vi "Start Personal Log.vi"(8 "error in (no error)":errorcluster, 11 "Father of all uServices in":refnum<class "Father of all uServices.lvclass">) -> (0 "error out":errorcluster, 3 "Father of all uServices out":refnum<class "Father of all uServices.lvclass">)   [LabVIEW 2026, in "TALOS.lvlib" / "Father of all uServices.lvlib" / "Father of all uServices.lvclass"]
uses:
  Father of all uServices.lvclass
  C:/LabVIEW Code/TALOS/talos/Ancestor/Ancestor/Ancestor.lvclass
  Ancestor/Ancestor/Ancestor.lvclass/Ancestor.ctl
  Father of all uServices.lvclass/Father of all uServices.ctl
  Support VIs/Generate Error.vi
  FGV/Error Memory/Get Error Description.vi
  Support VIs/Get PC name.vi
  Support VIs/Get Class Name.vi
  <vilib>/Utility/error.llb/Clear Errors.vi
  FGV/Error Memory/Error Memory Core.vi
  <vilib>/AdvancedString/Delimited String to 1D String Array.vi
  <vilib>/AdvancedString/Delimited String to 1D String Array (string).vi
  Support VIs/Circus Root Path.vi
  FGV/Error Memory/Error Crt Lvl checker.vi
  FGV/Error Memory/Error Memory Core.vi/40c8088d-b597-4017-91af-faa98e00292e.vi
  FGV/Error Memory/Error Memory Core.vi/d4a3ab98-063c-4e44-b43d-fbdcfe6c2be2.vi
  Support VIs/Global Memory.vi
  <vilib>/Utility/LVClass/Get LV Class Name.vi
  Support VIs/Is in Packed Library.vi
  Support VIs/TALOS Root path.vi
  Support VIs/Read CSV worksheet.vi
  Support VIs/Global Constants.vi
  <vilib>/Utility/error.llb/General Error Handler.vi
  Support VIs/Error Log.vi
  Ancestor/Ancestor/Ancestor.lvclass
  <vilib>/Comparison/Equal/Equal Functor/Equal Functor.lvclass
  TALOS.lvlib
  Classes/Log/Log.lvclass
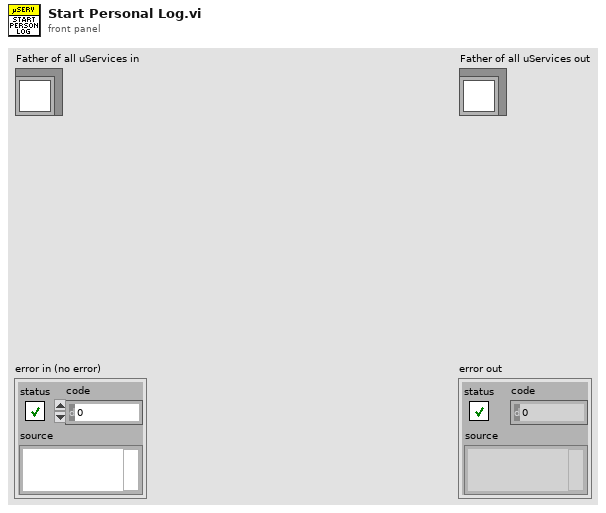
[diagram p1: front panel]
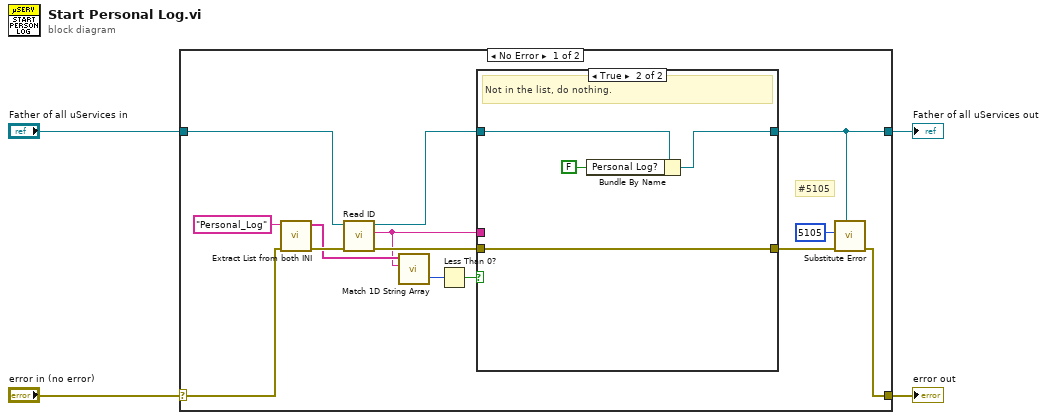
[diagram p0: block diagram]
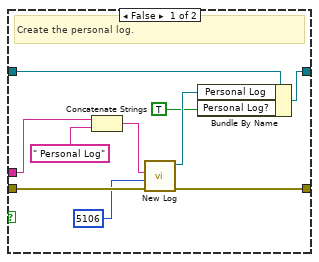
[diagram p2: hidden frame]
diagram:
  n1 = case shown="No Error" "error in (no error)" {
    selector: "error in (no error)" -> [w11 w34]
    tunnel: [w8 w34] -> w3
    tunnel: [w7 w33] -> w1
    tunnel: "Father of all uServices in" -> [w16 w33]
    frame No Error {
      # "#5105"
      n2 = call "Extract List from both INI.vi"("error in (no error)"=w11, "Parameter Name"="Personal_Log") -> ("error out"=w17:errorcluster, "Array"=w15:string[])  [unwired: 8 in]
      n3 = call "Read ID.vi"("error in (no error)"=w17, "Ancestor in"=w16) -> ("error out"=w10:errorcluster, "ID"=w5:string, "Ancestor out"=w12:refnum<class "Father of all uServices.lvclass">)  [unwired: 7 in]
      n4 = call <vilib>:"Match 1D String Array.vi"("Pattern"=w5, "Strings"=w15) -> ("index of element"=w14:i32)  [unwired: 2 in, 1 out]
      n5 = Less Than 0?(x=w14) -> (x < 0?=w13:bool)
      n6 = case shown="True" w13 {
        tunnel: [w21 w30] -> w7
        tunnel: w12 -> [w22 w32]
        tunnel: w10 -> [w28 w31]
        tunnel: [w27 w31] -> w9
        tunnel: w5 -> [w24 _]
        frame False {
          # "Create the personal log."
          n7 = Concatenate Strings(w24, " Personal Log") -> (w23:string)
          n8 = call "New Log.vi"("error in (no error)"=w28, "Specific Error Code"=5106, "Name"=w23) -> ("error out"=w27:errorcluster, "Log out"=w20:refnum<class "Log.lvclass">)  [unwired: 7 in]
          n9 = Bundle By Name(cluster=w22, "Personal Log"=w20, "Personal Log?"=TRUE) -> (w21:refnum<class "Father of all uServices.lvclass">)
        }
        frame True {
          # "Not in the list, do nothing."
          n10 = Bundle By Name(cluster=w32, "Personal Log?"=FALSE) -> (w30:refnum<class "Father of all uServices.lvclass">)
        }
      }
      n11 = call "Substitute Error.vi"("LabVIEW Object"=w7, "error in (no error)"=w9, "Error Code"=5105) -> ("error out"=w8:errorcluster)  [unwired: 8 in]
    }
    frame Error {
    }
  }
  "error out" <- w3
  "Father of all uServices out" <- w1
